vi "Tools_System Memory Status.vi"(8 "error in (no error)":errorcluster) -> (0 "error out":errorcluster, 1 "Free memory (%)":dbl, 2 "Free memory (MB)":dbl, 3 "Total memory (MB)":dbl, 5 "Memory Used (MB)":string)   [LabVIEW 2021]
uses:
  kernel32.dll
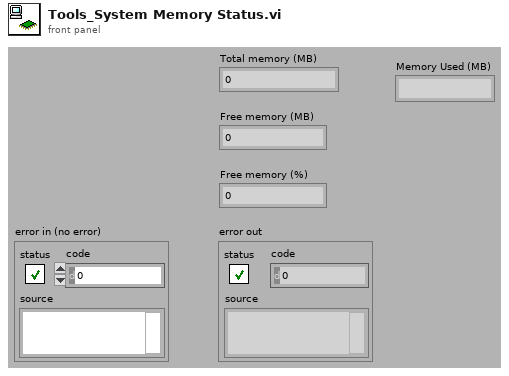
[diagram p1: front panel]
types:
  T1 = cluster{"dwLength":u32, "dwMemoryLoad":u32, "ullTotalPhys":u64, "ullAvailPhys":u64, "ullTotalPageFile":u64, "ullAvailPageFile":u64, "ullTotalVirtual":u64, "ullAvailVirtual":u64, "ullAvailExtendedVirtual":u64}
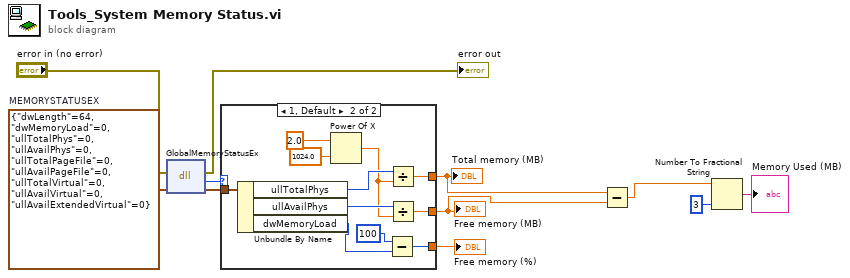
[diagram p0: block diagram]
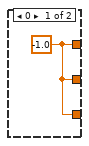
[diagram p2: hidden frame]
diagram:
  w8 = T1 {"dwLength"=64, "dwMemoryLoad"=0, "ullTotalPhys"=0, "ullAvailPhys"=0, "ullTotalPageFile"=0, "ullAvailPageFile"=0, "ullTotalVirtual"=0, "ullAvailVirtual"=0, "ullAvailExtendedVirtual"=0}  # MEMORYSTATUSEX
  n1 = dll-call lib="kernel32.dll" fn="GlobalMemoryStatusEx"(error in="error in (no error)", w8) -> (error out=→"error out":errorcluster, "return type"=w9:i32, w10:T1)  [unwired: 2 in, 1 out]
  n2 = case shown="1, Default" w9 {
    tunnel: w10 -> [_ w23]
    tunnel: [w12 w13] -> w11
    tunnel: [w12 w17] -> w5
    tunnel: [w12 w16] -> w4
    frame 0 {
      w12 = -1.0
    }
    frame 1, Default {
      n3 = Unbundle By Name(w23) -> ("ullTotalPhys"=w20:u64, "ullAvailPhys"=w19:u64, "dwMemoryLoad"=w14:u32)
      n4 = Power Of X(1:1024.0 ("x"), 2:2.0 ("y")) -> (0:w18:dbl)
      n5 = Subtract(x=u32 100, y=w14) -> (x-y=w13:u32)
      n6 = Divide(x=w20, y=w18) -> (x/y=w17:dbl)
      n7 = Divide(x=w19, y=w18) -> (x/y=w16:dbl)
    }
  }
  "Free memory (%)" <- w11
  "Free memory (MB)" <- w4
  "Total memory (MB)" <- w5
  n8 = Subtract(x=w5, y=w4) -> (x-y=w3:dbl)
  n9 = Number To Fractional String(number=w3, precision (6)=i16 3) -> (F-format string=→"Memory Used (MB)":string)  [unwired: 2 in]
